vi "Fuzzy-Input.vi"(0 "Slide in":refnum<vi>, 1 "Positive Lower Limit [Fixed]":dbl, 2 "Slide Refnum 4":refnum<vi>, 3 "Max Err":dbl, 4 "Slide Refnum 5":refnum<vi>, 6 "Slide Refnum 3":refnum<vi>, 7 "Zero Lower Limit":dbl, 8 "Min Intersection":dbl, 9 "Negative Upper Limit [Fixed]":dbl, 10 "Slide Refnum in":refnum<vi>, 11 "Zero Upper Limit":dbl, 12 "Min Err":dbl, 13 "Zero Medium Limit [Fixed]":dbl) -> (14 "Array":cluster{dbl[], dbl[]}[](array[cluster]))   [LabVIEW 2016]
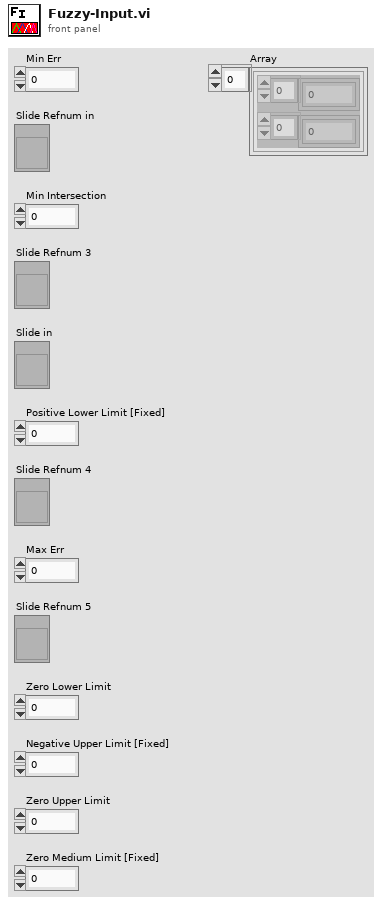
[diagram p1: front panel]
types:
  T1 = enum8{"Enabled", "Disabled", "Disabled and Grayed Out"}
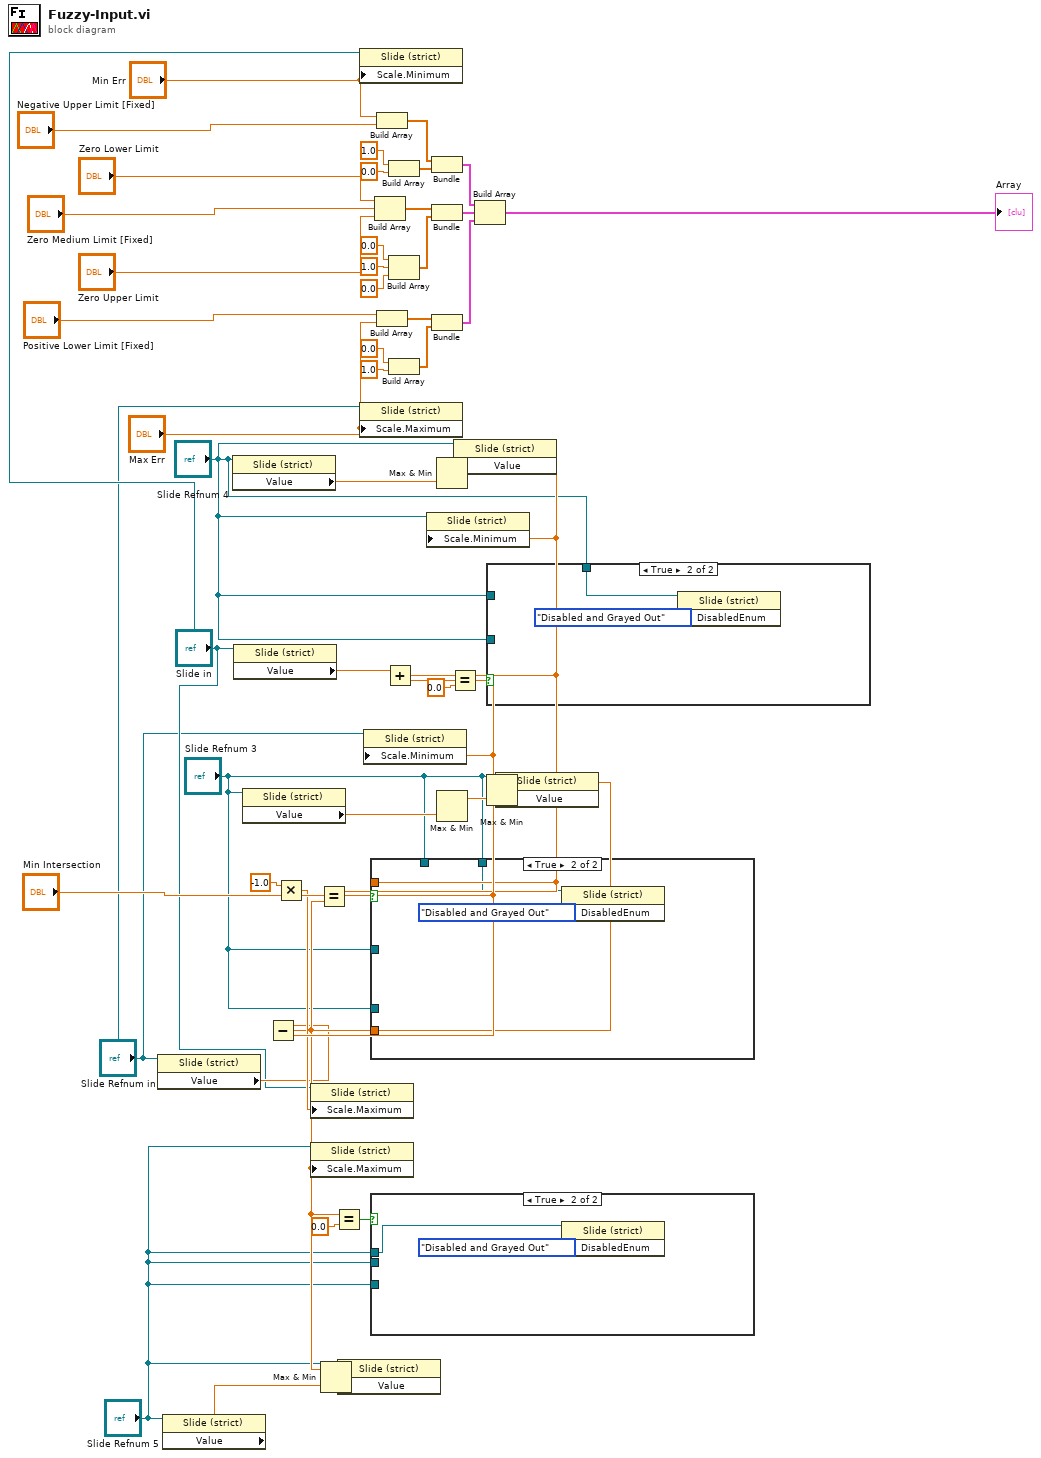
[diagram p0: block diagram]
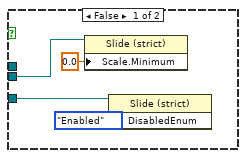
[diagram p2: hidden frame]
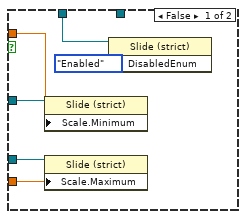
[diagram p3: hidden frame]
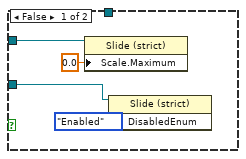
[diagram p4: hidden frame]
diagram:
  n1 = property on="Property Node" class="Slide (strict)"(reference="Slide Refnum in") -> ("Value"=w30:dbl)  [unwired: 1 in, 2 out]
  n2 = property on="Property Node" class="Slide (strict)"(reference="Slide Refnum 5") -> ("Value"=w38:dbl)  [unwired: 1 in, 2 out]
  n3 = property on="Property Node" class="Slide (strict)"(reference="Slide Refnum 4") -> ("Value"=w32:dbl)  [unwired: 1 in, 2 out]
  n4 = property on="Property Node" class="Slide (strict)"(reference="Slide in") -> ("Value"=w33:dbl)  [unwired: 1 in, 2 out]
  n5 = property on="Property Node" class="Slide (strict)"(reference="Slide Refnum 3") -> ("Value"=w31:dbl)  [unwired: 1 in, 2 out]
  n6 = Subtract(x=w30, y="Min Intersection") -> (x-y=w41:dbl)
  n7 = Multiply(x=-1.0, y="Min Intersection") -> (x*y=w47:dbl)
  n8 = property on="Property Node" class="Slide (strict)"(reference="Slide in", "Scale.Maximum"=w47) -> ()  [unwired: 1 in, 2 out]
  n9 = property on="Property Node" class="Slide (strict)"(reference="Slide Refnum 5", "Scale.Maximum"=w41) -> ()  [unwired: 1 in, 2 out]
  n10 = Max & Min(x=w41, y=w38) -> (min(x,y)=w39:dbl)  [unwired: 1 out]
  n11 = Equal?(x=w41, y=0.0) -> (x = y?=w43:bool)
  n12 = property on="Property Node" class="Slide (strict)"(reference="Slide Refnum 5", "Value"=w39) -> ()  [unwired: 1 in, 2 out]
  n13 = property on="Property Node" class="Slide (strict)"(reference="Slide in", "Scale.Minimum"="Min Err") -> ()  [unwired: 1 in, 2 out]
  n14 = property on="Property Node" class="Slide (strict)"(reference="Slide Refnum in", "Scale.Maximum"="Max Err") -> ()  [unwired: 1 in, 2 out]
  n15 = property on="Property Node" class="Slide (strict)"(reference="Slide Refnum in", "Scale.Minimum"="Min Intersection") -> ()  [unwired: 1 in, 2 out]
  n16 = case shown="True" w43 {
    tunnel: "Slide Refnum 5" -> [w50 _]
    tunnel: "Slide Refnum 5" -> [w49 _]
    tunnel: "Slide Refnum 5" -> [_ w53]
    frame False {
      n17 = property on="Property Node" class="Slide (strict)"(reference=w49, "Scale.Minimum"=0.0 ("Scale.Range:Minimum")) -> ()  [unwired: 1 in, 2 out]
      n18 = property on="Property Node" class="Slide (strict)"(reference=w50, "DisabledEnum"=T1."Enabled" ("Disabled")) -> ()  [unwired: 1 in, 2 out]
    }
    frame True {
      n19 = property on="Property Node" class="Slide (strict)"(reference=w53, "DisabledEnum"=T1."Disabled and Grayed Out" ("Disabled")) -> ()  [unwired: 1 in, 2 out]
    }
  }
  n20 = Build Array("Zero Lower Limit", "Zero Medium Limit [Fixed]", "Zero Upper Limit") -> (w17:dbl[])
  n21 = Build Array("Min Err", "Negative Upper Limit [Fixed]") -> (w9:dbl[])
  n22 = Build Array("Positive Lower Limit [Fixed]", "Max Err") -> (w24:dbl[])
  n23 = Add(x=w33, y="Min Intersection") -> (x+y=w40:dbl)
  n24 = Equal?(x=w40, y=w41) -> (x = y?=w37:bool)
  n25 = case shown="True" w37 {
    tunnel: w40 -> [w59 _]
    tunnel: w41 -> [w58 _]
    tunnel: "Slide Refnum 3" -> [w57 _]
    tunnel: "Slide Refnum 3" -> [w56 _]
    tunnel: "Slide Refnum 3" -> [w55 _]
    tunnel: "Slide Refnum 3" -> [_ w61]
    frame False {
      n26 = property on="Property Node" class="Slide (strict)"(reference=w56, "Scale.Minimum"=w59) -> ()  [unwired: 1 in, 2 out]
      n27 = property on="Property Node" class="Slide (strict)"(reference=w55, "Scale.Maximum"=w58) -> ()  [unwired: 1 in, 2 out]
      n28 = property on="Property Node" class="Slide (strict)"(reference=w57, "DisabledEnum"=T1."Enabled" ("Disabled")) -> ()  [unwired: 1 in, 2 out]
    }
    frame True {
      n29 = property on="Property Node" class="Slide (strict)"(reference=w61, "DisabledEnum"=T1."Disabled and Grayed Out" ("Disabled")) -> ()  [unwired: 1 in, 2 out]
    }
  }
  n30 = Build Array(1.0 ("element"), 0.0 ("element")) -> (w10:dbl[])
  n31 = Build Array(0.0 ("element"), 1.0 ("element"), 0.0 ("element")) -> (w18:dbl[])
  n32 = Build Array(0.0 ("element"), 1.0 ("element")) -> (w25:dbl[])
  n33 = property on="Property Node" class="Slide (strict)"(reference="Slide Refnum 4", "Scale.Minimum"=w40) -> ()  [unwired: 1 in, 2 out]
  n34 = Bundle(w9, w10) -> (w19:cluster{dbl[], dbl[]})  [unwired: 1 in]
  n35 = Bundle(w17, w18) -> (w20:cluster{dbl[], dbl[]})  [unwired: 1 in]
  n36 = Bundle(w24, w25) -> (w27:cluster{dbl[], dbl[]})  [unwired: 1 in]
  n37 = Max & Min(x=w40, y=w32) -> (max(x,y)=w34:dbl)  [unwired: 1 out]
  n38 = Max & Min(x=w40, y=w31) -> (max(x,y)=w29:dbl)  [unwired: 1 out]
  n39 = Equal?(x=w40, y=0.0) -> (x = y?=w36:bool)
  n40 = property on="Property Node" class="Slide (strict)"(reference="Slide Refnum 4", "Value"=w34) -> ()  [unwired: 1 in, 2 out]
  n41 = Build Array(w19, w20, w27) -> (→"Array":cluster{dbl[], dbl[]}[])
  n42 = case shown="True" w36 {
    tunnel: "Slide Refnum 4" -> [w64 _]
    tunnel: "Slide Refnum 4" -> [w63 _]
    tunnel: "Slide Refnum 4" -> [_ w67]
    frame False {
      n43 = property on="Property Node" class="Slide (strict)"(reference=w64, "Scale.Maximum"=0.0 ("Scale.Range:Maximum")) -> ()  [unwired: 1 in, 2 out]
      n44 = property on="Property Node" class="Slide (strict)"(reference=w63, "DisabledEnum"=T1."Enabled" ("Disabled")) -> ()  [unwired: 1 in, 2 out]
    }
    frame True {
      n45 = property on="Property Node" class="Slide (strict)"(reference=w67, "DisabledEnum"=T1."Disabled and Grayed Out" ("Disabled")) -> ()  [unwired: 1 in, 2 out]
    }
  }
  n46 = Max & Min(x=w41, y=w29) -> (min(x,y)=w28:dbl)  [unwired: 1 out]
  n47 = property on="Property Node" class="Slide (strict)"(reference="Slide Refnum 3", "Value"=w28) -> ()  [unwired: 1 in, 2 out]
